vi "PID (DBL Array) Obsolete.vi"(6 "reinitialize? (F)":bool, 7 "output range":cluster{"output high":dbl, "output low":dbl}[](array[cluster])=[{"output high"=100.0, "output low"=-100.0}] {"output low" format="%.2f"; "output high" format="%.2f"}, 8 "dt (s)":dbl=-1.0 format="%.3f", 9 "PID gains":T1(array[cluster])=[{"proportional gain (Kc)"=1.0, "integral time (Ti, min)"=0.01, "derivative time (Td, min)"=0.0}] {"derivative time (Td, min)" format="%.3f"; "integral time (Ti, min)" format="%.3f"; "proportional gain (Kc)" format="%.3f"}, 10 "process variable":dbl[](array[numeric])=[0.0] format="%.2f", 11 "setpoint":dbl[](array[numeric])=[0.0] format="%.2f") -> (0 "dt out (s)":dbl format="%.3f", 3 "output":dbl[](array[numeric]) format="%.2f")   [LabVIEW 2020, in "NI_PID_pid.lvlib"]
doc: "PID algorithm for simple PID applications or high speed control applications that require an efficient algorithm. PID algorithm features control output range limiting with integrator anti-windup and bumpless controller output for PID gain changes."
uses:
  NI_PID_pid.lvlib
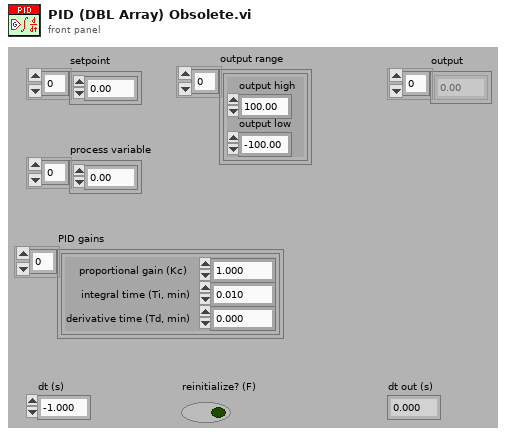
[diagram p1: front panel]
types:
  T1 = cluster{"proportional gain (Kc)":dbl, "integral time (Ti, min)":dbl, "derivative time (Td, min)":dbl}[]
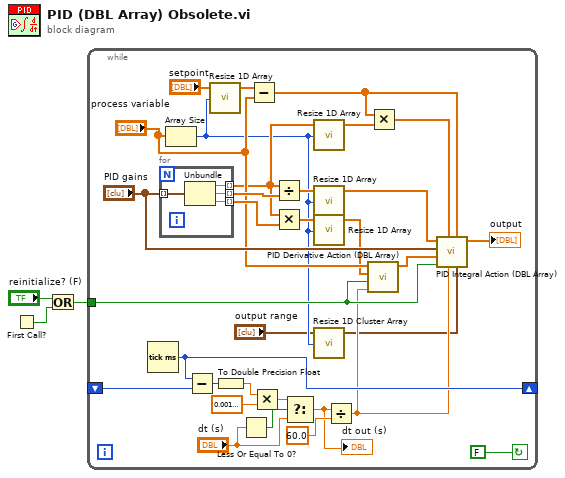
[diagram p0: block diagram]
diagram:
  n1 = First Call?() -> (First Call?: T/F=w3:bool)
  n2 = Or(x="reinitialize? (F)", y=w3) -> (x .or. y?=w2:bool)
  n3 = while {
    tunnel: w2 -> [w21]
    shift-left: _ -> [w29]
    shift-right: [w28] -> _
    stop <- FALSE continue-if-true
    n4 = Tick Count (ms)() -> (millisecond timer value=w28:u32)
    n5 = for {
      tunnel: [w39] -> w26 mode=indexing
      tunnel: [w38] -> w25 mode=indexing
      tunnel: [w37] -> w13 mode=indexing
      tunnel: "PID gains" -> [w36] mode=indexing
      n6 = Unbundle(w36) -> ("proportional gain (Kc)"=w37:dbl, "integral time (Ti, min)"=w39:dbl, "derivative time (Td, min)"=w38:dbl)
    }
    n7 = Array Size(array="process variable") -> (size(s)=w7:i32)
    n8 = Subtract(x=w28, y=w29) -> (x-y=w33:u32)
    n9 = call "Resize 1D Array.vi"("array size"=w7, "input array"="setpoint") -> ("output array"=w14:dbl[])  [unwired: 3 out]
    n10 = To Double Precision Float(number=w33) -> (double precision float=w32:dbl)
    n11 = Less Or Equal To 0?(x="dt (s)") -> (x <= 0?=w30:bool)
    n12 = Subtract(x=w14, y="process variable") -> (x-y=w24:dbl[])
    n13 = Multiply(x=w32, y=0.0010000000474974513) -> (x*y=w31:dbl)
    n14 = Divide(x=w13, y=w26) -> (x/y=w11:dbl[])
    n15 = Multiply(x=w13, y=w25) -> (x*y=w8:dbl[])
    n16 = Select(t=w31, s=w30, f="dt (s)") -> (s? t:f=w4:dbl)
    "dt out (s)" <- w4
    n17 = call "Resize 1D Array.vi"("array size"=w7, "input array"=w13) -> ("output array"=w12:dbl[])  [unwired: 3 out]
    n18 = call "Resize 1D Array.vi"("array size"=w7, "input array"=w11) -> ("output array"=w10:dbl[])  [unwired: 3 out]
    n19 = call "Resize 1D Array.vi"("array size"=w7, "input array"=w8) -> ("output array"=w9:dbl[])  [unwired: 3 out]
    n20 = call "Resize 1D Cluster Array.vi"("array size"=w7, "input array"="output range") -> ("output array"=w6:cluster{"output high":dbl, "output low":dbl}[])  [unwired: 3 out]
    n21 = Divide(x=w4, y=60.0) -> (x/y=w20:dbl)
    n22 = call "PID Derivative Action (DBL Array).vi"("dt (min)"=w20, "initialize (F)"=w21, "Kd"=w9, "process variable"="process variable") -> ("derivative action"=w22:dbl[])  [unwired: 3 out]
    n23 = Multiply(x=w24, y=w12) -> (x*y=w23:dbl[])
    n24 = call "PID Integral Action (DBL Array).vi"("output range"=w6, "error"=w24, "dt (min)"=w20, "proportional action"=w23, "initialize (F)"=w21, "derivative action"=w22, "PID gains"="PID gains", "Ki"=w10) -> ("output"=→"output":dbl[])  [unwired: 3 out]
  }
